vi "AH_SRQHalt.vi"(7 "timeout":u32=25000, 8 "error in (no error)":errorcluster, 10 "Data Cluster In":T1 {"GUI Data Cluster"."SBR" format="%08b"}, 11 "Config Cluster In":T3) -> (0 "error out":errorcluster {"code" format="%x"}, 1 "SRQ Timed Out":bool, 2 "Data Cluster Out":T1 {"GUI Data Cluster"."SBR" format="%08b"}, 3 "Configuration Cluster Out":T3={"General"={"Config.ini"=path "", "Default Logging Path"=path ""}, "Hardware"={"AHC VISA COM"="", "Measure Rate (1/s)"=0, "Global T VAR"="", "Global B VAR"=""}, "Operation"={"Operation Mode"=enum."Idle-Off", "Status"="", "NewLog?"=FALSE}})   [LabVIEW 2021]
uses:
  Config_Cluster.ctl
  Mode_Enum.ctl
  Data_Cluster.ctl
  Measurement_Cluster.ctl
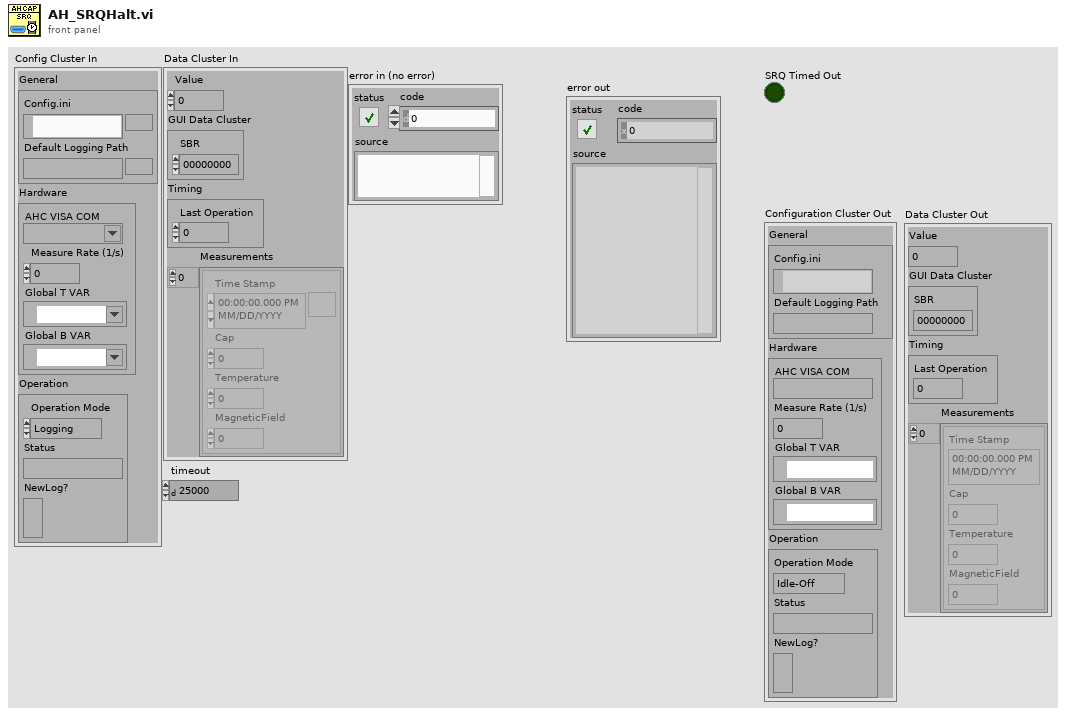
[diagram p1: front panel]
types:
  T1 = typedef "Data_Cluster.ctl" = cluster{"Value":dbl, "GUI Data Cluster":cluster{"SBR":u16}, "Timing":cluster{"Last Operation":dbl}, "Measurements":T2[]}
  T2 = typedef "Measurement_Cluster.ctl" = cluster{"Time Stamp":timestamp, "Cap":dbl, "Temperature":dbl, "MagneticField":dbl}
  T3 = typedef "Config_Cluster.ctl" = cluster{"General":cluster{"Config.ini":path, "Default Logging Path":path}, "Hardware":cluster{"AHC VISA COM":refnum<visa-resource-name>, "Measure Rate (1/s)":i32, "Global T VAR":refnum<k21>, "Global B VAR":refnum<k21>}, "Operation":cluster{"Operation Mode":T4, "Status":string, "NewLog?":bool}}
  T4 = typedef "Mode_Enum.ctl" = enum16{"Logging", "Idle-Off", "Idle"}
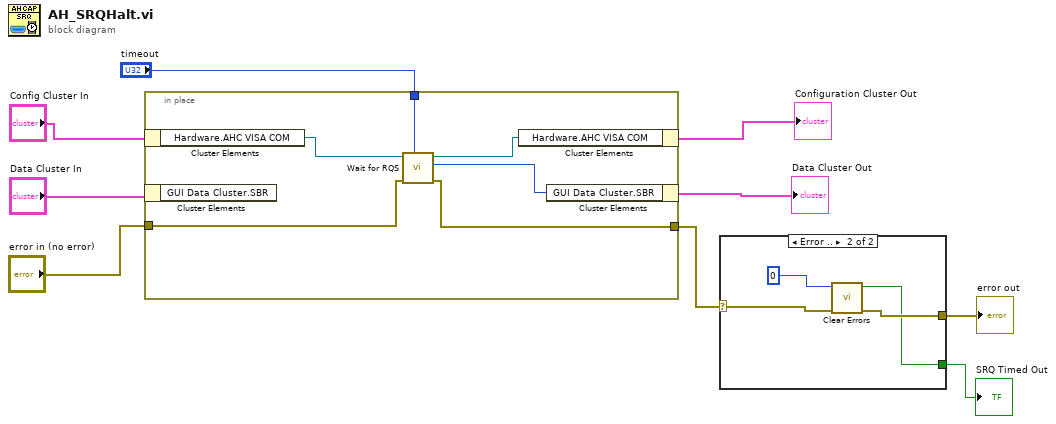
[diagram p0: block diagram]
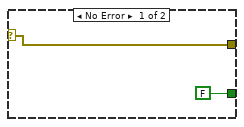
[diagram p2: hidden frame]
diagram:
  n1 = in-place {
    in-place-border: "error in (no error)" -> [w12]
    in-place-border: [w11] -> w3
    in-place-border: "timeout" -> [w10]
    n2 = in-place-cluster #1("Config Cluster In") -> ("Hardware.AHC VISA COM"=w15:refnum<visa-resource-name>)
    n3 = in-place-cluster #2("Data Cluster In") -> ()  [unwired: 1 out]
    n4 = call <vilib>:"Wait for RQS.vi"("timeout (25000 ms)"=w10, "error in (no error)"=w12, "VISA resource name"=w15) -> ("error out"=w11:errorcluster, "status byte"=w13:u16, "VISA resource name out"=w14:refnum<visa-resource-name>)  [unwired: 6 in]
    n5 = in-place-cluster #1("Hardware.AHC VISA COM"=w14) -> (→"Configuration Cluster Out":T3)
    n6 = in-place-cluster #2("GUI Data Cluster.SBR"=w13) -> (→"Data Cluster Out":T1)
  }
  n7 = case shown="Error .." w3 {
    selector: w3 -> [w17 w21]
    tunnel: [w17 w20] -> w2
    tunnel: [FALSE w19] -> w1
    frame No Error {
    }
    frame Error {
      n8 = call <vilib>:"Clear Errors.vi"("error in (no error)"=w21, "specific error code to clear (0: all)"=0) -> ("error out"=w20:errorcluster, "specific error cleared?"=w19:bool)  [unwired: 4 in]
    }
  }
  "error out" <- w2
  "SRQ Timed Out" <- w1
